vi "UI_VISA.vi"() -> ()   [LabVIEW 2021]
uses:
  <vilib>/Instr/_visa.llb/VISA Configure Serial Port (Instr).vi
panel:
  in  "termination char\n(0xA = '\\n' = LF)":u8=10 format="%.0x"
  in  "K_omega":dbl=0.8
  in  "K_theta":dbl=0.4
  in  "Theta_ref":dbl(slide)=-0.4255319148936181 scale=-20.0..20.0
  out "u2":dbl=1060.0
  out "u2":dbl(graph)=1060.0
  out "u1":dbl(graph)=1059.0
  out "u1":dbl=1059.0
  out "Omega":dbl(graph)=-0.0
  out "Omega":dbl=-0.0
  out "Theta":dbl(graph)=0.8
  out "Theta":dbl=0.8
  out "Input String":string="0.80,-0.00,1059,1060\r\n"
  in  "VISA resource name":refnum<visa-resource-name>="COM5"
  in  "Stop Button":bool
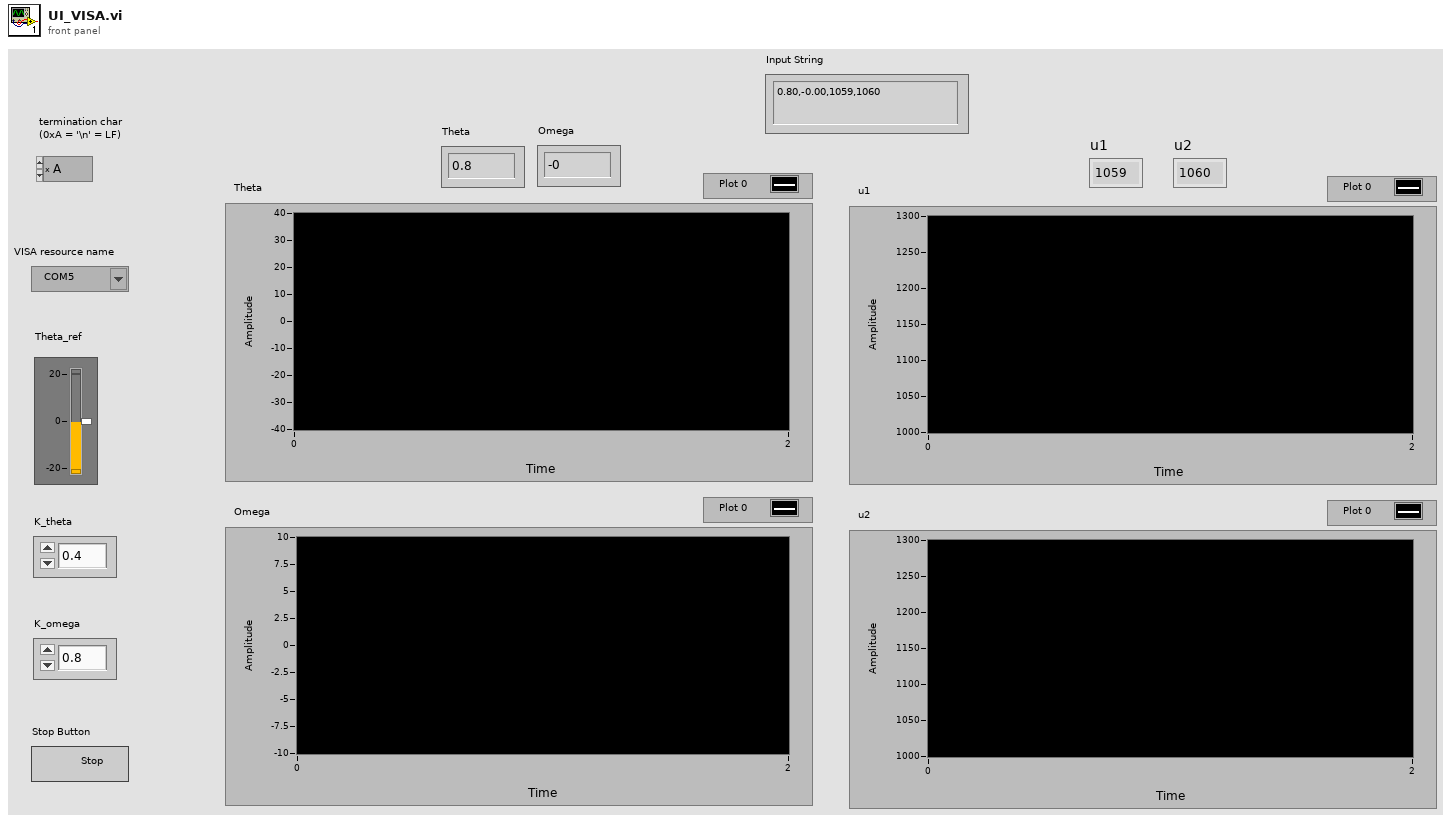
[diagram p1: front panel]
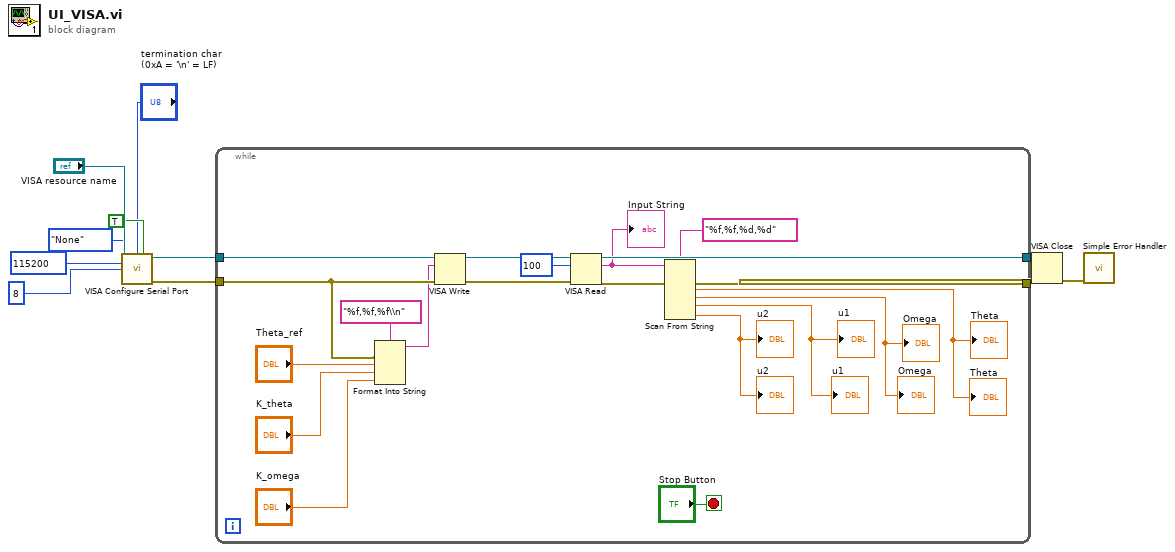
[diagram p0: block diagram]
diagram:
  n1 = call-poly "VISA Configure Serial Port"("VISA resource name"="VISA resource name", "termination char\n(0xA = '\\n' = LF)"="termination char\n(0xA = '\\n' = LF)", "Enable Termination\nChar (T)"=TRUE ("Enable Termination\nChar (T)"), "baud rate (9600)"=u32 115200, "data bits (8)"=u16 8, "parity (0:none)"=enum16{"None", "Odd", "Even", "Mark", "Space"}."None") -> ("VISA resource name out"=w10:refnum<visa-resource-name>, "error out"=w8:errorcluster)  [unwired: 8 in]
  n2 = while {
    tunnel: w10 -> [w20]
    tunnel: w8 -> [w14]
    tunnel: [w29] -> w7
    tunnel: [w24] -> w6
    stop <- "Stop Button" stop-if-true
    n3 = Format Into String(format string="%f,%f,%f\\n", error in=w14, "Theta_ref", "K_theta", "K_omega") -> (resulting string=w12:string)  [unwired: 1 in, 1 out]
    n4 = VISA Write(VISA resource name=w20, write buffer=w12, error in (no error)=w14) -> (VISA resource name out=w19:refnum<visa-resource-name>, error out=w18:errorcluster)  [unwired: 1 out]
    n5 = VISA Read(VISA resource name=w19, byte count=u32 100, error in (no error)=w18) -> (VISA resource name out=w29:refnum<visa-resource-name>, read buffer=w27:string, error out=w25:errorcluster)  [unwired: 1 out]
    "Input String" <- w27
    n6 = Scan From String(format string="%f,%f,%d,%d", input string=w27, error in=w25) -> (error out=w24:errorcluster, output 1=→"Theta" →"Theta":dbl, output 2=→"Omega" →"Omega":dbl, output 3=→"u1" →"u1":dbl, output 4=→"u2" →"u2":dbl)  [unwired: 5 in, 2 out]
  }
  n7 = VISA Close(VISA resource name=w7, error in (no error)=w6) -> (error out=w5:errorcluster)
  n8 = call <vilib>:"Simple Error Handler.vi"("error in (no error)"=w5) -> ()  [unwired: 4 in, 5 out]
